vi "check_island.vi"(1 "start_square":T1, 2 "tour_in_progress":T1[](array[typedef]), 3 "chessboard":T2[][](array[typedef])) -> (0 "T = an island was found":bool)   [LabVIEW 2020, in "core.lvlib"]
uses:
  core.lvlib
  core_data/chessboard_index.ctl
  core_data/chess_square.ctl
  core_data/neighbour_square.ctl
  core_data/core_data.lvlib
panel:
  # "Development\ncontrols/indicators useful for development and testing, but which are not outputs of the VI"
  # "Input\nInputs to the VI"
  # "Output\nOutputs of the VI"
  # "Description\n\nBlank VI with error handling case. \n\nSummarize the use of this VI in this space."
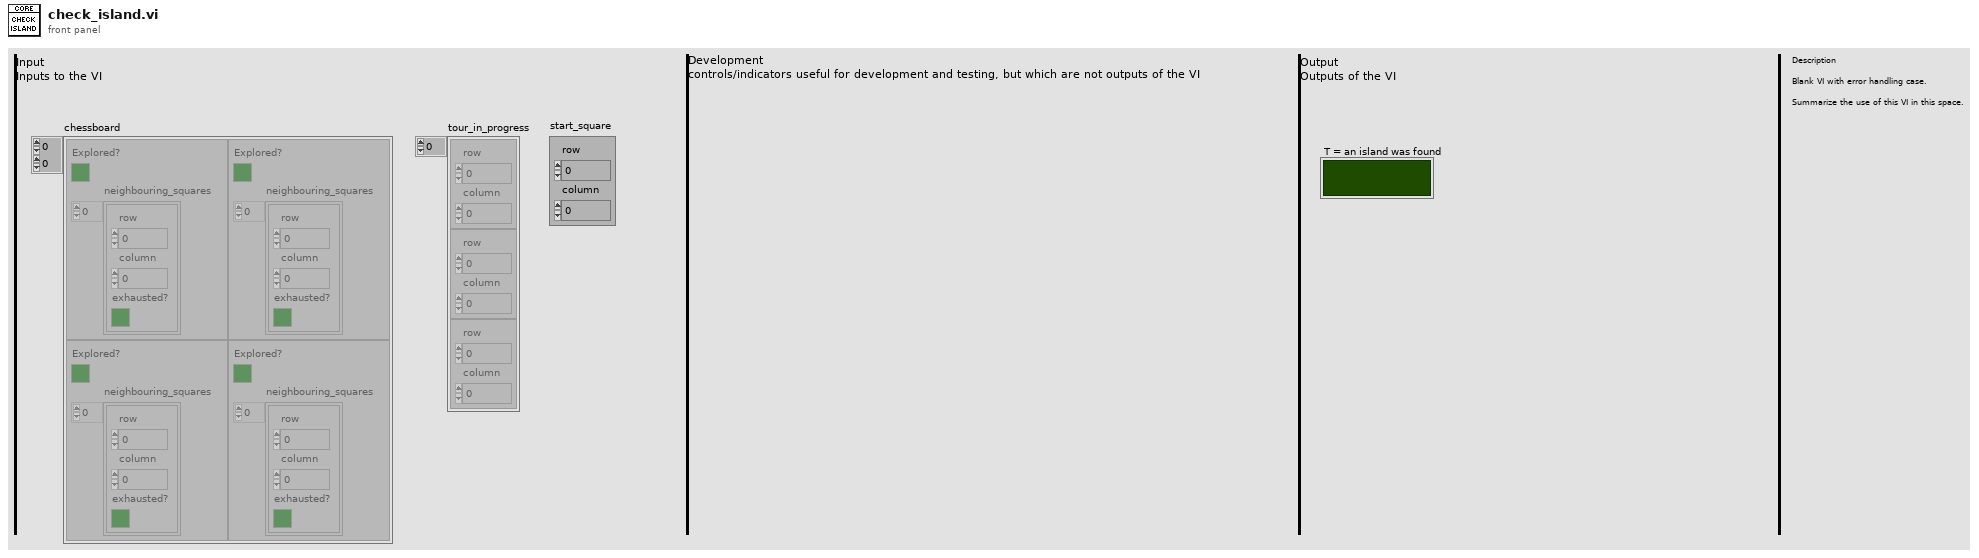
[diagram p1: front panel]
types:
  T1 = typedef "core.lvlib/core_data.lvlib/chessboard_index.ctl" = cluster{"row":u8, "column":u8}
  T2 = typedef "core.lvlib/core_data.lvlib/chess_square.ctl" = cluster{"Explored?":bool, "neighbouring_squares":T3[]}
  T3 = typedef "core.lvlib/core_data.lvlib/neighbour_square.ctl" = cluster{"row":u8, "column":u8, "exhausted?":bool}
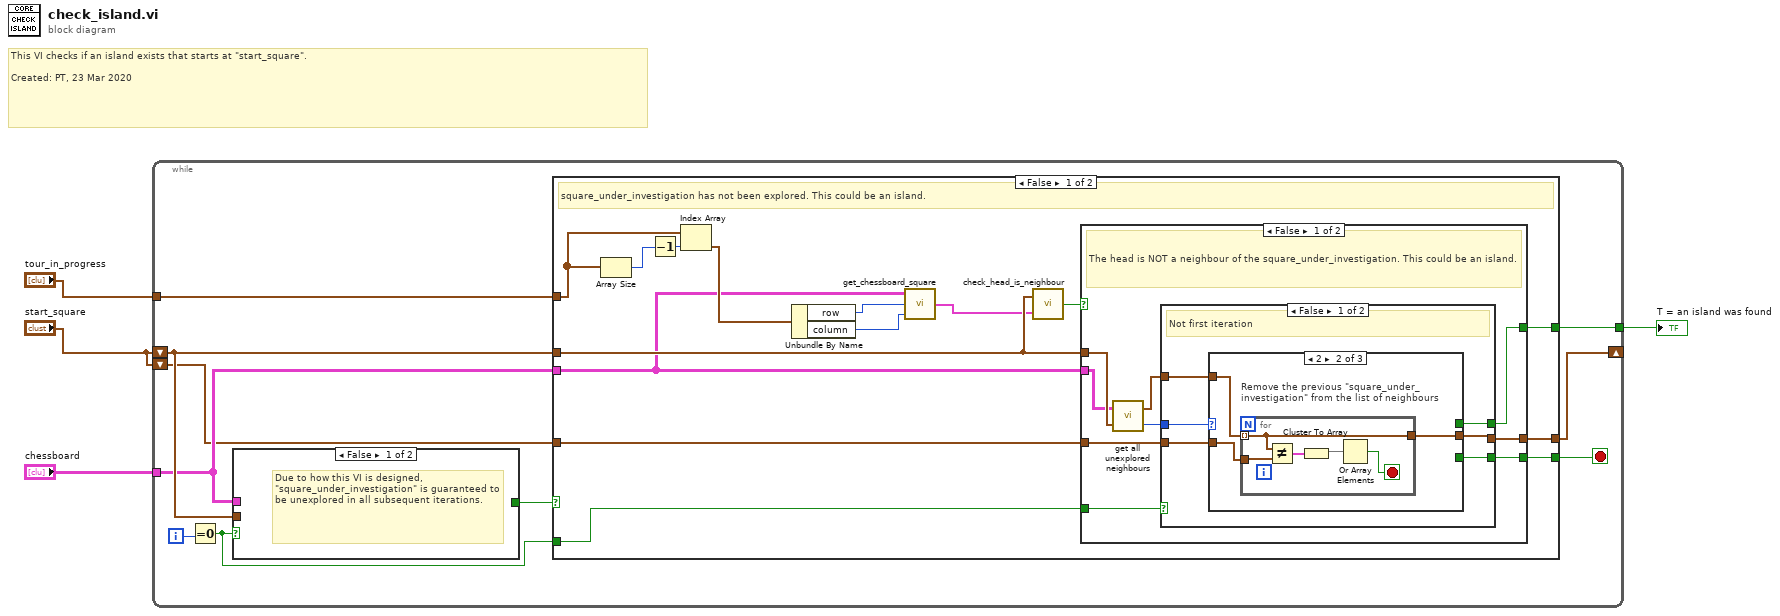
[diagram p0: block diagram]
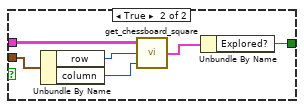
[diagram p2: hidden frame]
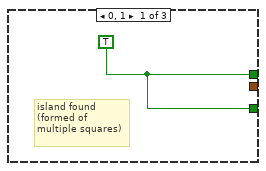
[diagram p3: hidden frame]
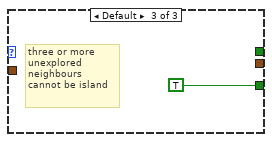
[diagram p4: hidden frame]
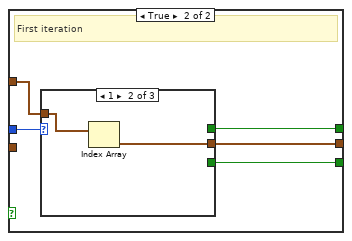
[diagram p5: hidden frame]
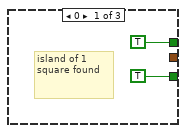
[diagram p6: hidden frame]
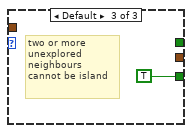
[diagram p7: hidden frame]
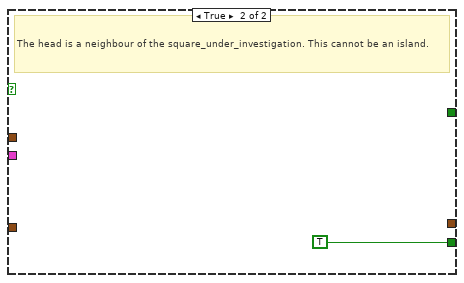
[diagram p8: hidden frame]
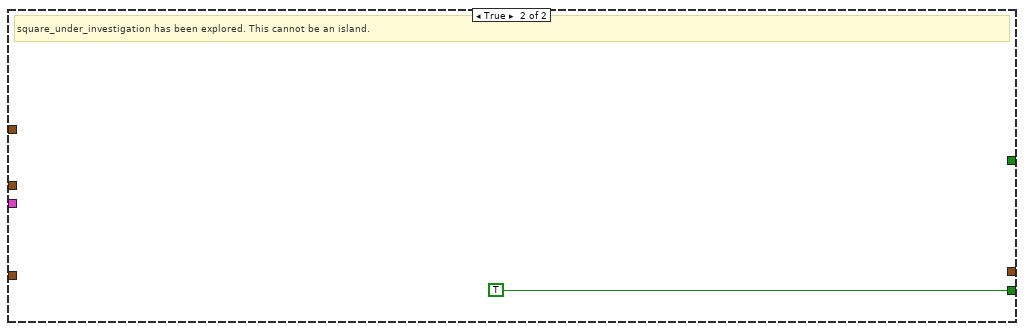
[diagram p9: hidden frame]
diagram:
  # "This VI checks if an island exists that starts at \"start_square\".\n\nCreated: PT, 23 Mar 2020"
  n1 = while {
    shift-right: [w7] -> _
    shift-left: "start_square" -> [w12]
    tunnel: [w13] -> w4
    tunnel: "chessboard" -> [w9]
    shift-left: "start_square" -> [w6]
    tunnel: "tour_in_progress" -> [w5]
    i -> [w10]
    stop <- w14 stop-if-true
    n2 = Equal To 0?(x=w10) -> (x = 0?=w8:bool)
    n3 = case shown="False" w8 {
      tunnel: w9 -> [_ w20]
      tunnel: w12 -> [_ w19]
      tunnel: [_ w15] -> w11
      frame False {
        # "Due to how this VI is designed,\n\"square_under_investigation\" is guaranteed to be unexplored in all subsequent iterations."
      }
      frame True {
        n4 = Unbundle By Name(w19) -> ("row"=w18:u8, "column"=w17:u8)
        n5 = call "get_chessboard_square.vi"("column"=w17, "row"=w18, "chessboard"=w20) -> ("chessboard_square"=w16:T2)
        n6 = Unbundle By Name(w16) -> ("Explored?"=w15:bool)
      }
    }
    n7 = case shown="False" w11 {
      tunnel: [w34 TRUE] -> w14
      tunnel: [w33 _] -> w13
      tunnel: w12 -> [w32 _]
      tunnel: w9 -> [w22 _]
      tunnel: w8 -> [w31 _]
      tunnel: [w30 _] -> w7
      tunnel: w6 -> [w29 _]
      tunnel: w5 -> [w23 _]
      frame False {
        # "square_under_investigation has not been explored. This could be an island."
        n8 = Array Size(array=w23) -> (size(s)=w28:i32)
        n9 = Decrement(x=w28) -> (x-1=w27:i32)
        n10 = Index Array(array=w23, index=w27) -> (element=w26:T1)
        n11 = Unbundle By Name(w26) -> ("row"=w25:u8, "column"=w24:u8)
        n12 = call "get_chessboard_square.vi"("column"=w24, "row"=w25, "chessboard"=w22) -> ("chessboard_square"=w21:T2)
        n13 = call "check_head_is_neighbour.vi"("head (square knight is sitting on)"=w21, "square to check"=w32) -> ("T = the HEAD is a neighbour"=w35:bool)
        n14 = case shown="False" w35 {
          tunnel: [w40 TRUE] -> w34
          tunnel: [w39 _] -> w33
          tunnel: w32 -> [w44 _]
          tunnel: w22 -> [w43 _]
          tunnel: w31 -> [w42 _]
          tunnel: [w37 _] -> w30
          tunnel: w29 -> [w36 _]
          frame False {
            # "The head is NOT a neighbour of the square_under_investigation. This could be an island."
            n15 = call "get all unexplored neighbours.vi"("square (chessboard index)"=w44, "chessboard"=w43) -> ("no. of unexplored neighbours"=w41:i32, "unexplored neighbours"=w38:T1[])
            n16 = case shown="False" w42 {
              tunnel: w41 -> [w50 w65]
              tunnel: [w48 w64] -> w40
              tunnel: [w49 w63] -> w39
              tunnel: w38 -> [w47 w62]
              tunnel: [w45 w61] -> w37
              tunnel: w36 -> [w46 _]
              frame False {
                # "Not first iteration"
                n17 = case shown="2" w50 {
                  tunnel: [w51 _ _] -> w49
                  tunnel: [w51 _ TRUE] -> w48
                  tunnel: w47 -> [_ w54 _]
                  tunnel: w46 -> [_ w53 _]
                  tunnel: [_ w52 _] -> w45
                  frame 0, 1 {
                    w51 = TRUE
                    # "island found (formed of multiple squares)"
                  }
                  frame 2 {
                    n18 = for "Remove the previous \"square_under_investigation\" from the list of neighbours" {
                      tunnel: w54 -> [w55] mode=indexing
                      tunnel: w53 -> [w59]
                      tunnel: [w55] -> w52
                      stop <- w56 stop-if-true
                      n19 = Not Equal?(x=w55, y=w59) -> (x != y?=w58:cluster{"row":bool, "column":bool})
                      n20 = Cluster To Array(cluster=w58) -> (array=w57:bool[])
                      n21 = Or Array Elements(Boolean array=w57) -> (logical OR=w56:bool)
                    }
                  }
                  frame Default {
                    # "three or more unexplored neighbours\ncannot be island"
                  }
                }
              }
              frame True {
                # "First iteration"
                n22 = case shown="1" w65 {
                  tunnel: [TRUE _ _] -> w63
                  tunnel: [TRUE _ TRUE] -> w64
                  tunnel: w62 -> [_ w69 _]
                  tunnel: [_ w68 _] -> w61
                  frame 0 {
                    # "island of 1 square found"
                  }
                  frame 1 {
                    n23 = Index Array(array=w69) -> (element=w68:T1)  [unwired: 1 in]
                  }
                  frame Default {
                    # "two or more unexplored neighbours\ncannot be island"
                  }
                }
              }
            }
          }
          frame True {
            # "The head is a neighbour of the square_under_investigation. This cannot be an island."
          }
        }
      }
      frame True {
        # "square_under_investigation has been explored. This cannot be an island."
      }
    }
  }
  "T = an island was found" <- w4
